vi "Read State.vi"(8 "error in (no error)":errorcluster, 11 "Module in":refnum<class "Module.lvclass">) -> (0 "error out":errorcluster, 2 "State":T1, 3 "Module out":refnum<class "Module.lvclass">)   [LabVIEW 2014, in "Module.lvclass"]
uses:
  Module.lvclass
  Module_State.ctl
  Module.lvclass/Module.ctl
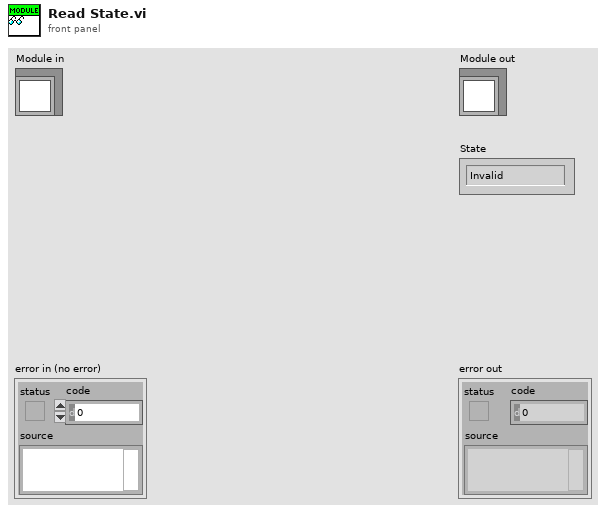
[diagram p1: front panel]
types:
  T1 = typedef "Module.lvclass/Module_State.ctl" = enum16{"Invalid", "Error", "InMemory", "Waiting", "Running"}
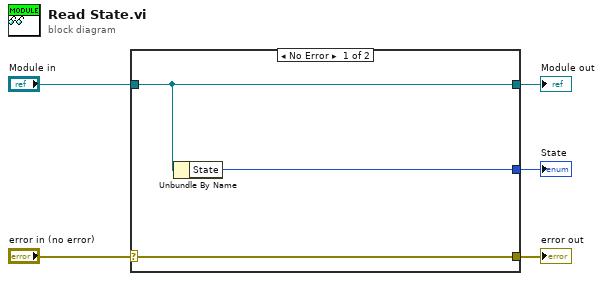
[diagram p0: block diagram]
diagram:
  n1 = case shown="No Error" "error in (no error)" {
    selector: "error in (no error)" -> [w8 w9]
    tunnel: [w8 w9] -> w4
    tunnel: [w7 w10] -> w2
    tunnel: "Module in" -> [w7 w10]
    tunnel: [w6 _] -> w1
    frame No Error {
      n2 = Unbundle By Name(w7) -> ("State"=w6:T1)
    }
    frame Error {
    }
  }
  "error out" <- w4
  "Module out" <- w2
  "State" <- w1
